vi "find data index.vi"(10 "string to locate":string, 11 "sorted list":T1) -> (3 "index":i32)   [LabVIEW 2013, in "tag bus.lvlib" / "binary search.lvlib"]
doc: "Searches through the sorted list for the string specified, and returns the associated data index."
uses:
  binary search.lvlib
  sorted list.ctl
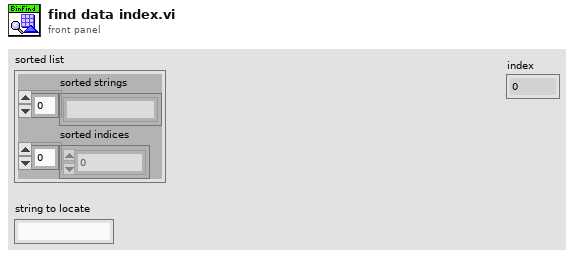
[diagram p1: front panel]
types:
  T1 = typedef "tag bus.lvlib/binary search.lvlib/sorted list.ctl" = cluster{"sorted strings":string[], "sorted indices":i32[]}
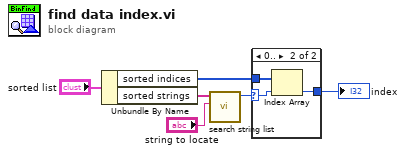
[diagram p0: block diagram]
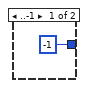
[diagram p2: hidden frame]
diagram:
  n1 = Unbundle By Name("sorted list") -> ("sorted indices"=w4:i32[], "sorted strings"=w5:string[])
  n2 = call "search string list.vi"("string to locate"="string to locate", "sorted strings"=w5) -> ("index"=w3:i32)  [unwired: 9 in]
  n3 = case shown="0.." w3 {
    selector: w3 -> [_ w9]
    tunnel: w4 -> [_ w10]
    tunnel: [-1 ("Numeric") w8] -> w2
    frame ..-1 {
    }
    frame 0.. {
      n4 = Index Array(array=w10, index=w9) -> (element=w8:i32)
    }
  }
  "index" <- w2
